vi "正面计算.vi"(0 "Image In":T1(plugin-control), 5 "图片处理效果参数":T13={"二值化参数"={"Lower value"=169.0, "Upper value"=255.0}, "形态学分析模式"=enum."Erode", "形态学 迭代次数"=3, "特殊分析-滤波"=[{"Measurement Parameter"=19, "Range Lower Value"=0.0, "Range Upper Value"=1400.0, "Range"=FALSE, "Measurement Type"=FALSE}], "特殊分析-移除/保留"=TRUE} {"特殊分析-滤波"."Measurement Parameter" items=["Center of Mass X", "Center of Mass Y", "First Pixel X", "First Pixel Y", "Bounding Rect Left", "Bounding Rect Top", "Bounding Rect Right", "Bounding Rect Bottom", "Max Feret Diameter Start X", "Max Feret Diameter Start Y", "Max Feret Diameter End X", "Max Feret Diameter End Y", "Max Horiz. Segment Length Left", "Max Horiz. Segment Length Right", "Max Horiz. Segment Length Row", "-", "Bounding Rect Width", "Bounding Rect Height", "Bounding Rect Diagonal", "Perimeter", "Convex Hull Perimeter", "Holes' Perimeter", "Max Feret Diameter", "Equivalent Ellipse Major Axis", "Equivalent Ellipse Minor Axis", "Equivalent Ellipse Minor Axis (Feret)", "Equivalent Rect Long Side", "Equivalent Rect Short Side", "Equivalent Rect Diagonal", "Equivalent Rect Short Side (Feret)", "Average Horiz. Segment Length", "Average Vert. Segment Length", "Hydraulic Radius", "Waddel Disk Diameter", "-", "Area", "Holes' Area", "Particle & Holes' Area", "Convex Hull Area", "Image Area", "-", "Number of Holes", "Number of Horiz. Segments", "Number of Vert. Segments", "-", "Orientation", "Max Feret Diameter Orientation", "-", "% Area/Image Area", "% Area/(Particle & Holes' Area)", "Ratio of Equivalent Ellipse Axes", "Ratio of Equivalent Rect Sides", "-", "Elongation Factor", "Compactness Factor", "Heywood Circularity Factor", "Type Factor", "-", "Sum X", "Sum Y", "Sum XX", "Sum XY", "Sum YY", "Sum XXX", "Sum XXY", "Sum XYY", "Sum YYY", "-", "Moment of Inertia XX", "Moment of Inertia XY", "Moment of Inertia YY", "Moment of Inertia XXX", "Moment of Inertia XXY", "Moment of Inertia XYY", "Moment of Inertia YYY", "Norm. Moment of Inertia XX", "Norm. Moment of Inertia XY", "Norm. Moment of Inertia YY", "Norm. Moment of Inertia XXX", "Norm. Moment of Inertia XXY", "Norm. Moment of Inertia XYY", "Norm. Moment of Inertia YYY", "Hu Moment 1", "Hu Moment 2", "Hu Moment 3", "Hu Moment 4", "Hu Moment 5", "Hu Moment 6", "Hu Moment 7"]}, 7 "定位分析参数设定":T12={"是否启动图片分析"=FALSE, "定位圆环ROI"={"Center X"=1247, "Center Y"=1475, "Inner Radius"=0, "Outer Radius"=400, "Start Angle"=0.0, "End Angle"=0.0}, "圆环Options "={"Process"=enum."Get First Edge", "Step Size"=10, "Max Pixel Radius"=3}, "Options (Find Circular)"={"Search  Direction"=1, "Edge Options"={"Edge Polarity"=0, "Kernel Size"=3, "Width"=3, "Minimum Edge Strength"=178.0, "Interpolation Type"=enum."Bilinear Fixed", "Data Processing Method"=enum."Average"}, "Show Search Area"=FALSE, "Show Search Lines"=FALSE, "Show Edges Found"=FALSE, "Show Result"=FALSE, "Search Area Color"=65280, "Search Lines Color"=255, "Edge Locations Color"=16776960, "Result Color"=16711680, "Overlay Group Name"=""}} {"Options (Find Circular)"."Search  Direction" items=["Outside to Inside", "Inside to Outside"]; "Options (Find Circular)"."Edge Options"."Edge Polarity" items=["All Edges", "Rising Edges", "Falling Edges"]; "Options (Find Circular)"."Edge Options"."Minimum Edge Strength" format="%.2f"; "Options (Find Circular)"."Edge Options"."Width" step=2; "Options (Find Circular)"."Edge Options"."Kernel Size" step=2; "定位圆环ROI"."End Angle" min=-90.0 max=90.0 step=1.0 format="%.2f"; "定位圆环ROI"."Start Angle" min=-90.0 max=90.0 step=1.0 format="%.2f"; "定位圆环ROI"."Center X" scale=0.0..1024.0}, 9 "分析参数设定":T9={"溢出距离下限"="", "溢出距离上限"="", "像素分辨率"="", "Search Direction "=enum."Annulus Outer To Inner", "Curve Extraction "={"Extraction Mode"=0, "Edge Threshold"=75, "Edge Filter Size"=0, "Min Length"=25, "Search Step Size"=15, "Max Endpoint Gap"=10, "Subpixel"=TRUE}, "Contour Selection "=enum."Closest To Search Start", "Curve Connection "=[{"Match Constraints"=0, "Min"=1.0, "Max"=12.0}], "Kernel Width "=5, "Curve Extraction 2 "={"Extraction Mode"=0, "Edge Threshold"=75, "Edge Filter Size"=0, "Min Length"=25, "Search Step Size"=15, "Max Endpoint Gap"=10, "Subpixel"=TRUE}, "Match Mode "={"Rotation"=FALSE, "Scale"=FALSE, "Occlusion"=FALSE}, "Smoothing Kernel "=0, "Template File Path "=path "C:/Users/hedongpo/Desktop/吕亚/Temp3.png", "Circle or Annulus"={"Center X"=1245, "Center Y"=1480, "Inner Radius"=238, "Outer Radius"=308, "Start Angle"=0.0, "End Angle"=0.0}} {"Circle or Annulus"."End Angle" min=-90.0 max=90.0 step=1.0 format="%.2f"; "Circle or Annulus"."Start Angle" min=-90.0 max=90.0 step=1.0 format="%.2f"; "Circle or Annulus"."Center X" scale=0.0..1024.0; "Curve Extraction"."Extraction Mode" items=["Normal", "Uniform Regions"]; "Curve Extraction"."Edge Filter Size" items=["Fine", "Normal", "Contour Tracing"]; "Curve Extraction"."Max Endpoint Gap" min=0; "Curve Extraction"."Search Step Size" min=1 max=255 step=1; "Curve Extraction"."Min Length" min=0; "Curve Extraction"."Edge Threshold" min=1 max=350 step=1; "Curve Connection"."Max" format="%.2f"; "Curve Connection"."Min" format="%.2f"; "Curve Connection"."Match Constraints" items=["Distance (pixel)", "Angle Difference (degrees)", "Connectivity Distance (pixel)", "Gradient Difference (degrees)"]; "Curve Extraction 2"."Extraction Mode" items=["Normal", "Uniform Regions"]; "Curve Extraction 2"."Edge Filter Size" items=["Fine", "Normal", "Contour Tracing"]; "Curve Extraction 2"."Max Endpoint Gap" min=0; "Curve Extraction 2"."Search Step Size" min=1 max=255 step=1; "Curve Extraction 2"."Min Length" min=0; "Curve Extraction 2"."Edge Threshold" min=1 max=350 step=1}, 11 "error in":errorcluster) -> (4 "Image Out":T1(plugin-control), 6 "Distances":T5(array[cluster]) {"Template Point"."Y" format="%.2f"; "Template Point"."X" format="%.2f"; "Target Point"."Y" format="%.2f"; "Target Point"."X" format="%.2f"}, 10 "Image Temple":T1, 15 "error out":errorcluster)   [LabVIEW 2017]
uses:
  <vilib>/vision/Measure.llb/Edge Options.ctl
  <vilib>/vision/Measure.llb/Edge Polarity.ctl
  <vilib>/vision/Contour.llb/IMAQ Contour Curve Extraction.ctl
  <vilib>/vision/Contour.llb/IMAQ Connect Range Setting.ctl
  <vilib>/vision/Image Controls.llb/IMAQ Image.ctl
  <vilib>/vision/Pattern Matching.llb/IMAQ Match Range Setting.ctl
  <vilib>/vision/NI_Vision_Development_Module.lvlib
panel:
  out "ROI Descriptor":T2 {"Contours"."Type" items=["No Selection", "Point", "Line", "Rectangle", "Oval", "Polygon", "Freehand Region", "Annulus", "Unused2", "Unused3", "Broken Line", "Freehand Line", "Rotated Rectangle"]}
  out "Coordinate System Out 2":T3 {"Measurement System"."Axis Reference" items=["Direct", "Indirect"]; "Measurement System"."Angle (deg)" format="%.2f"; "Measurement System"."Origin"."Y" format="%.2f"; "Measurement System"."Origin"."X" format="%.2f"; "Reference System"."Axis Reference" items=["Direct", "Indirect"]; "Reference System"."Angle (deg)" format="%.2f"; "Reference System"."Origin"."Y" format="%.2f"; "Reference System"."Origin"."X" format="%.2f"}
  out "Coordinate System Out":T3 {"Measurement System"."Axis Reference" items=["Direct", "Indirect"]; "Measurement System"."Angle (deg)" format="%.2f"; "Measurement System"."Origin"."Y" format="%.2f"; "Measurement System"."Origin"."X" format="%.2f"; "Reference System"."Axis Reference" items=["Direct", "Indirect"]; "Reference System"."Angle (deg)" format="%.2f"; "Reference System"."Origin"."Y" format="%.2f"; "Reference System"."Origin"."X" format="%.2f"}
  out "ROI Descriptor out 2":T2 {"Contours"."Type" items=["No Selection", "Point", "Line", "Rectangle", "Oval", "Polygon", "Freehand Region", "Annulus", "Unused2", "Unused3", "Broken Line", "Freehand Line", "Rotated Rectangle"]}
  out "输出簇":T4
  out "Center (Pixels) 2":cluster{"X":sgl, "Y":sgl}
  out "Valid?":bool
  out "Center (Pixels)":cluster{"X":sgl, "Y":sgl}
  out "ROI Descriptor out":T2 {"Contours"."Type" items=["No Selection", "Point", "Line", "Rectangle", "Oval", "Polygon", "Freehand Region", "Annulus", "Unused2", "Unused3", "Broken Line", "Freehand Line", "Rotated Rectangle"]}
  in  "File Path":path
  # "Range"
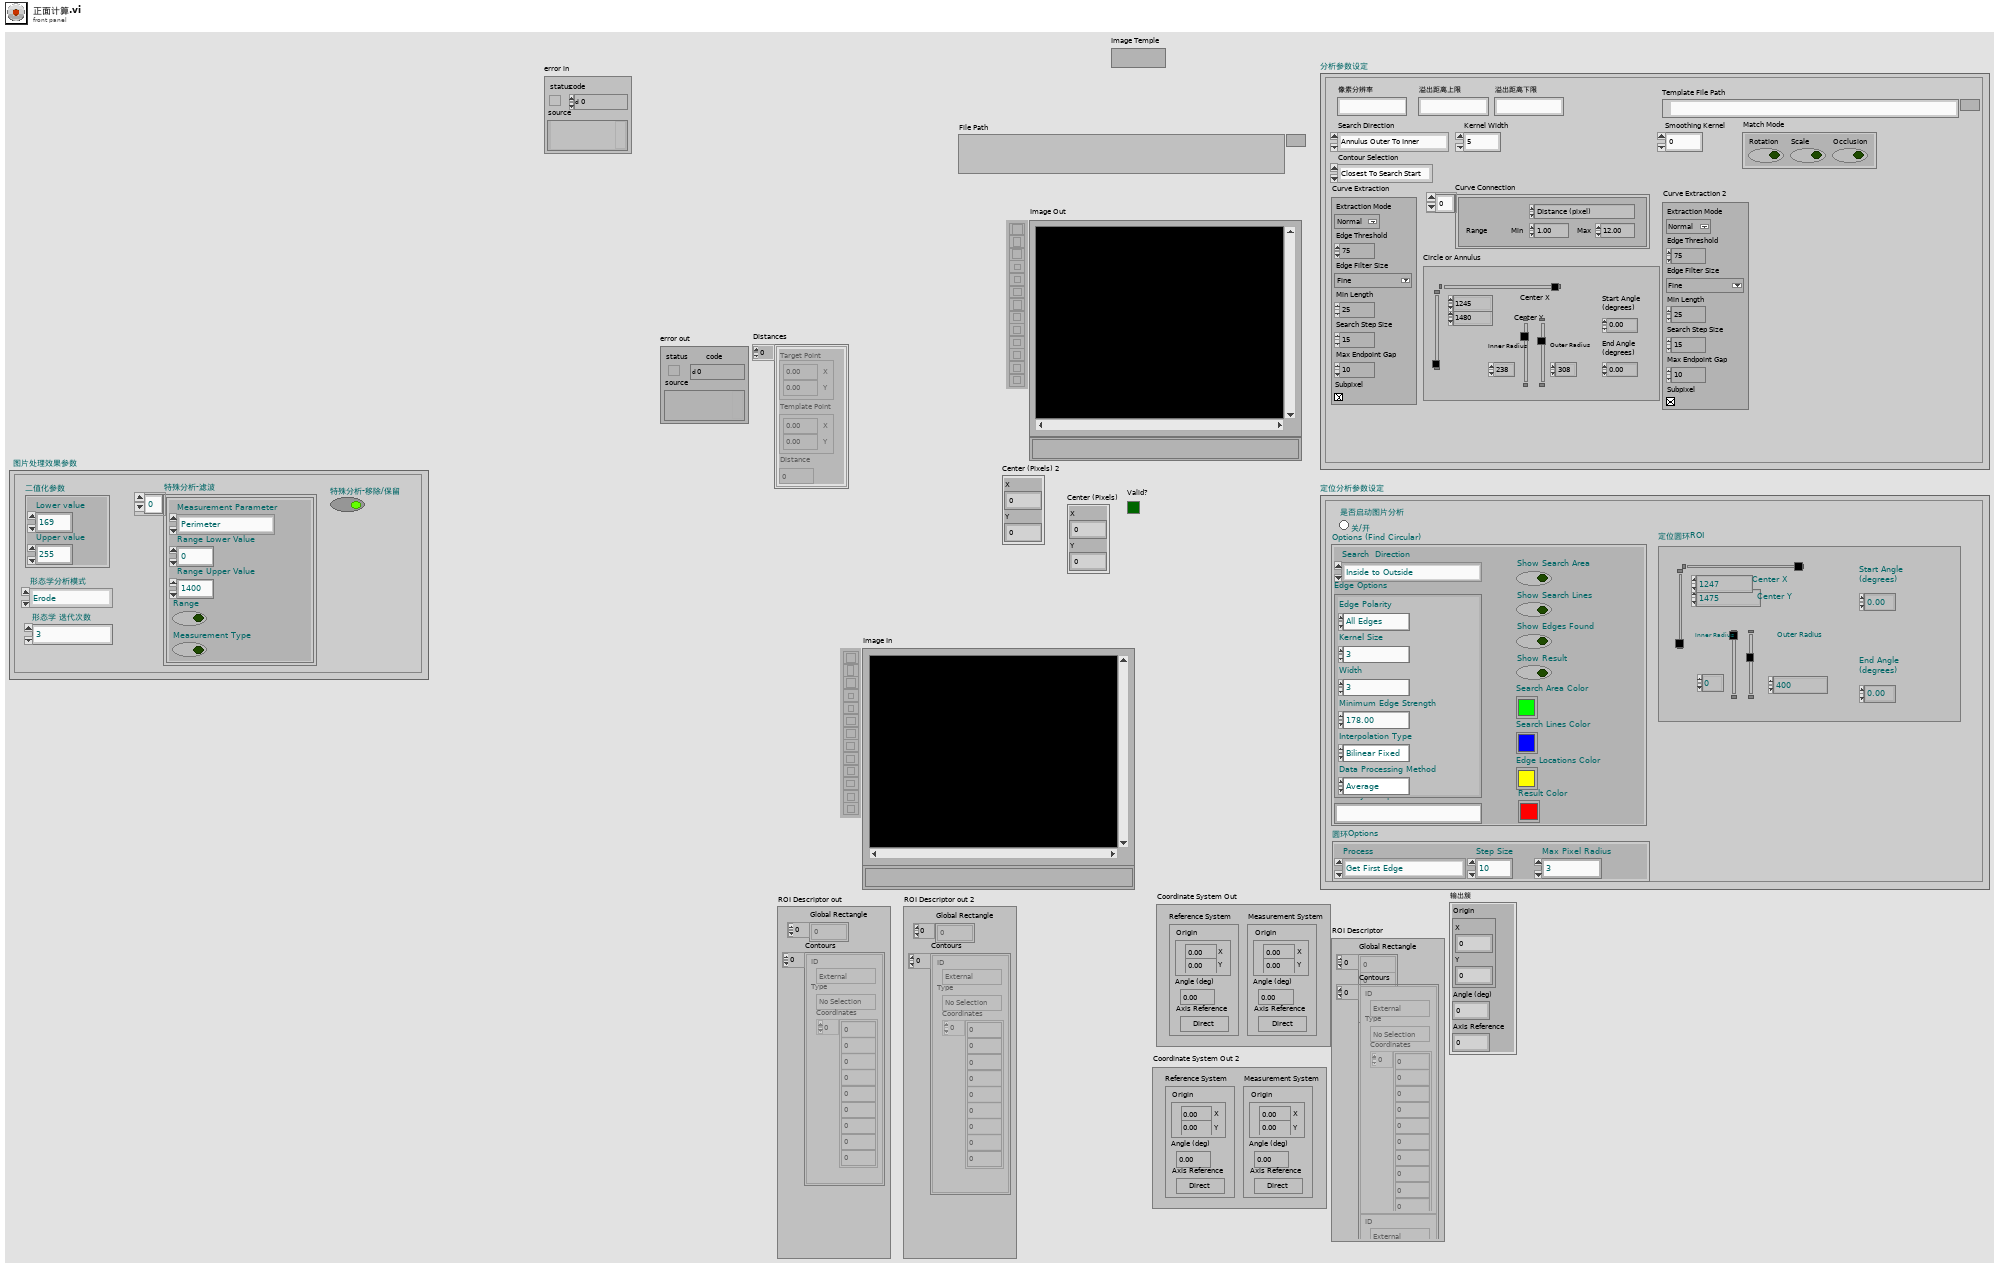
[diagram p1: front panel]
types:
  T1 = typedef "IMAQ Image.ctl" = refnum<image>
  T2 = typedef "ROI Descriptor" = cluster{"Global Rectangle":i32[], "Contours":cluster{"ID":enum32{"External", "Internal"}, "Type":u32, "Coordinates":i32[]}[]}
  T3 = typedef "IMAQ Coordinate System" = cluster{"Reference System":cluster{"Origin":cluster{"X":sgl, "Y":sgl}, "Angle (deg)":sgl, "Axis Reference":u32}, "Measurement System":cluster{"Origin":cluster{"X":sgl, "Y":sgl}, "Angle (deg)":sgl, "Axis Reference":u32}}
  T4 = cluster{"Origin":cluster{"X":sgl, "Y":sgl}, "Angle (deg)":sgl, "Axis Reference":u32}
  T5 = cluster{"Target Point":cluster{"X":dbl, "Y":dbl}, "Template Point":cluster{"X":dbl, "Y":dbl}, "Distance":dbl}[]
  T6 = typedef "IMAQ Contour Curve Extraction.ctl" = cluster{"Extraction Mode":u32, "Edge Threshold":i32, "Edge Filter Size":u32, "Min Length":i32, "Search Step Size":i32, "Max Endpoint Gap":i32, "Subpixel":bool}
  T7 = typedef "IMAQ Connect Range Setting.ctl" = cluster{"Match Constraints":u32, "Min":dbl, "Max":dbl}
  T8 = typedef "IMAQ Circle" = cluster{"Center X":i32, "Center Y":i32, "Inner Radius":i32, "Outer Radius":i32, "Start Angle":dbl, "End Angle":dbl}
  T9 = cluster{"溢出距离下限":string, "溢出距离上限":string, "像素分辨率":string, "Search Direction ":enum16{"Rect Left To Right", "Rect Right To Left", "Rect Top To Bottom", "Rect Bottom To Top", "Annulus Inner To Outer", "Annulus Outer To Inner", "Annulus Start Angle To End Angle", "Annulus End Angle To Start Angle"}, "Curve Extraction ":T6, "Contour Selection ":enum16{"Closest To Search Start", "Maximum Length", "Strongest Mean Gradient Change"}, "Curve Connection ":T7[], "Kernel Width ":u32, "Curve Extraction 2 ":T6, "Match Mode ":cluster{"Rotation":bool, "Scale":bool, "Occlusion":bool}, "Smoothing Kernel ":u32, "Template File Path ":path, "Circle or Annulus":T8}
  T10 = typedef "Edge Options.ctl" = cluster{"Edge Polarity":T11, "Kernel Size":u32, "Width":u32, "Minimum Edge Strength":sgl, "Interpolation Type":enum32{"Zero Order", "Bilinear", "Quadratic", "Cubic", "Bilinear Fixed"}, "Data Processing Method":enum32{"Average", "Median"}}
  T11 = typedef "Edge Polarity.ctl" = u32
  T12 = cluster{"是否启动图片分析":bool, "定位圆环ROI":T8, "圆环Options ":cluster{"Process":enum16{"Get First Edge", "Get First + Last Edge", "Get All Edges", "Get Best Edge"}, "Step Size":i32, "Max Pixel Radius":i32}, "Options (Find Circular)":cluster{"Search  Direction":u32, "Edge Options":T10, "Show Search Area":bool, "Show Search Lines":bool, "Show Edges Found":bool, "Show Result":bool, "Search Area Color":u32, "Search Lines Color":u32, "Edge Locations Color":u32, "Result Color":u32, "Overlay Group Name":string}}
  T13 = cluster{"二值化参数":cluster{"Lower value":sgl, "Upper value":sgl}, "形态学分析模式":enum32{"AutoM", "Close", "Dilate", "Erode", "Gradient", "Gradient out", "Gradient in", "Hit miss", "Open", "PClose", "POpen", "Thick", "Thin"}, "形态学 迭代次数":i32, "特殊分析-滤波":cluster{"Measurement Parameter":i32, "Range Lower Value":dbl, "Range Upper Value":dbl, "Range":bool, "Measurement Type":bool}[], "特殊分析-移除/保留":bool}
  T14 = cluster{"Overlay?":bool, "Color":u32, "Width":u32, "Maintain Width?":bool}
  T15 = cluster{"Search  Direction":u32, "Edge Options":T10, "Show Search Area":bool, "Show Search Lines":bool, "Show Edges Found":bool, "Show Result":bool, "Search Area Color":u32, "Search Lines Color":u32, "Edge Locations Color":u32, "Result Color":u32, "Overlay Group Name":string}
  T16 = typedef "IMAQ Match Range Setting.ctl" = cluster{"Match Constraints":u32, "Min":dbl, "Max":dbl}
  T17 = cluster{"Setup Data Item":u16, "Item Value":dbl}[]
  T18 = cluster{"Rotation":bool, "Scale":bool, "Occlusion":bool}
  T19 = enum16{"Closest To Search Start", "Maximum Length", "Strongest Mean Gradient Change"}
  T20 = enum16{"Rect Left To Right", "Rect Right To Left", "Rect Top To Bottom", "Rect Bottom To Top", "Annulus Inner To Outer", "Annulus Outer To Inner", "Annulus Start Angle To End Angle", "Annulus End Angle To Start Angle"}
  T21 = enum16{"Reset", "Update Coordinate System", "Get Coordinate System"}
  T22 = enum16{"Horizontal Motion", "Vertical Motion", "Horizontal and Vertical Motion", "Horizontal, Vertical and Angular Motion"}
  T23 = cluster{"Process":enum16{"Get First Edge", "Get First + Last Edge", "Get All Edges", "Get Best Edge"}, "Step Size":i32, "Max Pixel Radius":i32}
  T24 = cluster{"Global Rectangle":i32[], "Contours":cluster{"ID":enum32{"External", "Internal"}, "Type":u32, "Coordinates":i32[]}[]}
  T25 = cluster{"Measurement Parameter":i32, "Range Lower Value":dbl, "Range Upper Value":dbl, "Range":bool, "Measurement Type":bool}[]
  T26 = enum32{"AutoM", "Close", "Dilate", "Erode", "Gradient", "Gradient out", "Gradient in", "Hit miss", "Open", "PClose", "POpen", "Thick", "Thin"}
  T27 = typedef "Image Type" = u32
  T28 = cluster{"histogram":u32[], "Minimal Value":sgl, "Maximal Value":sgl, "Starting Value":sgl, "Interval Width":sgl, "Mean Value":sgl, "Standard  Variation":sgl, "Area (pixels)":i32}
  T29 = cluster{"Center (Pixels)":cluster{"X":sgl, "Y":sgl}, "Radius (Pixels)":dbl, "Center (Real-World)":cluster{"X":sgl, "Y":sgl}, "Radius (Real-World)":dbl, "Roundness (Real-World)":dbl, "Average Strength":dbl, "Average SNR (dB)":dbl}
  T30 = cluster{"Left":i32, "Top":i32, "Right":i32, "Bottom":i32}
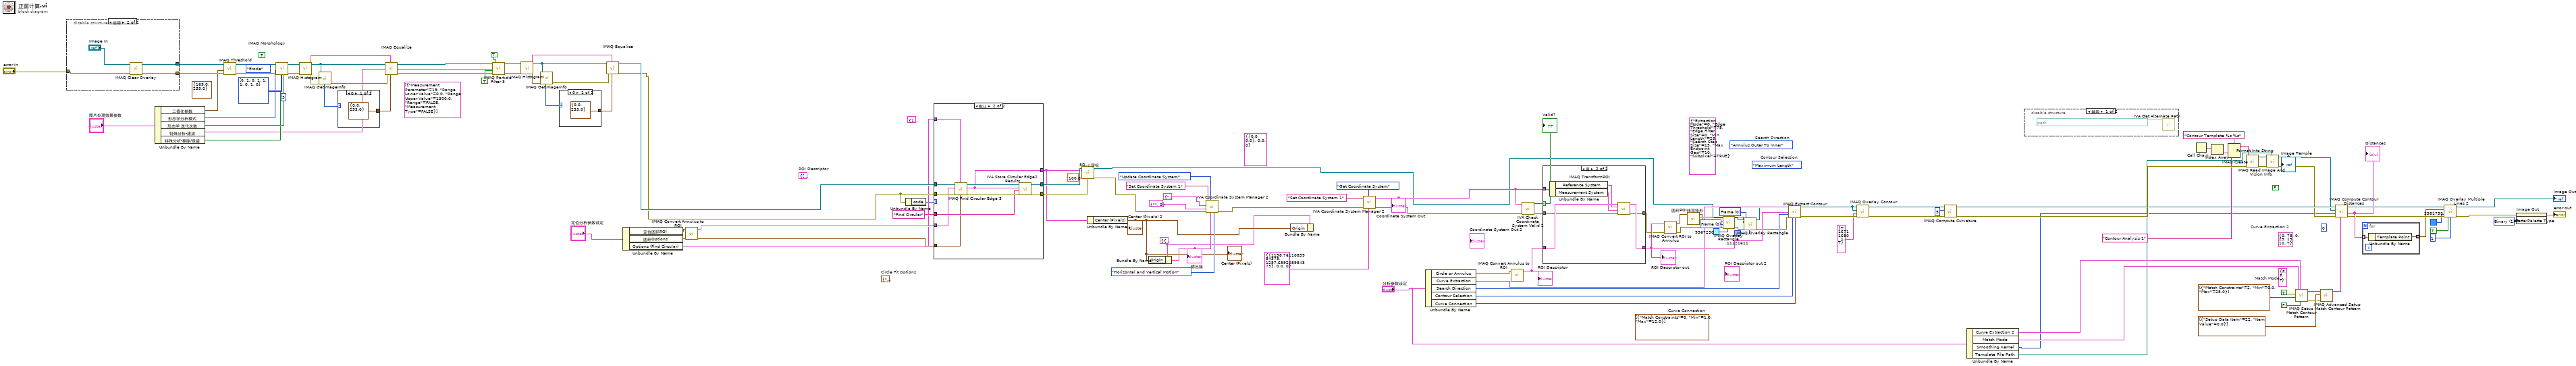
[diagram p0: block diagram]
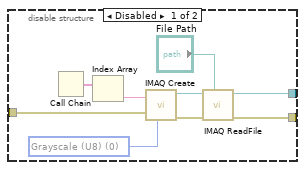
[diagram p2: hidden frame]
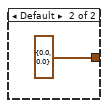
[diagram p6: hidden frame]
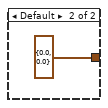
[diagram p7: hidden frame]
diagram:
  (unwired) FALSE
  w16 = u32 0 items=["Frame", "Fill", "Highlight"] ("Drawing Mode (Frame)")
  w19 = u32 0 items=["Frame", "Fill", "Highlight"] ("Drawing Mode (Frame)")
  (unwired) T6 {"Extraction Mode"=0, "Edge Threshold"=75, "Edge Filter Size"=0, "Min Length"=25, "Search Step Size"=15, "Max Endpoint Gap"=10, "Subpixel"=TRUE} ("Curve Extraction")
  (unwired) T15 {"Search  Direction"=1, "Edge Options"={"Edge Polarity"=0, "Kernel Size"=3, "Width"=3, "Minimum Edge Strength"=178.0, "Interpolation Type"=enum."Bilinear Fixed", "Data Processing Method"=enum."Average"}, "Show Search Area"=TRUE, "Show Search Lines"=TRUE, "Show Edges Found"=TRUE, "Show Result"=TRUE, "Search Area Color"=65280, "Search Lines Color"=255, "Edge Locations Color"=16776960, "Result Color"=16711680, "Overlay Group Name"=""} ("Options")
  (unwired) T6 {"Extraction Mode"=0, "Edge Threshold"=75, "Edge Filter Size"=0, "Min Length"=25, "Search Step Size"=15, "Max Endpoint Gap"=10, "Subpixel"=TRUE}  # Curve Extraction 2
  (unwired) T18 {"Rotation"=FALSE, "Scale"=FALSE, "Occlusion"=FALSE}  # Match Mode
  (unwired) u32 0 ("Smoothing Kernel")
  (unwired) T7[] [{"Match Constraints"=0, "Min"=1.0, "Max"=12.0}]  # Curve Connection
  (unwired) T19."Maximum Length"  # Contour Selection
  (unwired) T20."Annulus Outer To Inner"  # Search Direction
  (unwired) T4 {"Origin"={"X"=0.0, "Y"=0.0}, "Angle (deg)"=0.0, "Axis Reference"=0} ("Reference System")
  w2 = T4 {"Origin"={"X"=0.0, "Y"=0.0}, "Angle (deg)"=0.0, "Axis Reference"=0} ("Reference System")
  (unwired) T23 {"Process"=enum."Get First Edge", "Step Size"=20, "Max Pixel Radius"=3}  # Circle Fit Options
  (unwired) T24 {"Global Rectangle"=[683, 713, 1453, 1482], "Contours"=[{"ID"=enum."External", "Type"=7, "Coordinates"=[1067, 1097, 71, 384, 0, 0]}]}  # ROI Descriptor
  w96 = u32 1 items=["Grayscale", "Binary", "Gradient", "Rainbow", "Temperature", "User Defined", "Binary 16 Bit", "Gradient 16 Bit", "Rainbow 16 Bit", "Temperature 16 Bit", "User Defined 16 Bit"] ("Palette Type")
  (unwired) T25 [{"Measurement Parameter"=19, "Range Lower Value"=0.0, "Range Upper Value"=1300.0, "Range"=FALSE, "Measurement Type"=FALSE}] ("Selection Values")
  (unwired) 3 ("Number of iterations (1)")
  (unwired) T26."Erode" ("Operation")
  (unwired) FALSE ("Square/Hexa (Square)")
  (unwired) cluster{"Lower value":sgl, "Upper value":sgl} {"Lower value"=169.0, "Upper value"=255.0} ("Range")
  n1 = disable-structure shown="启用" {
    disable-tunnel: [w130 w131] -> w121
    disable-tunnel: "error in" -> [w127 w132]
    disable-tunnel: [w123 w133] -> w119
    frame Disabled {
      w124 = T27 0 items=["Grayscale (U8)", "Grayscale (I16)", "Grayscale (SGL)", "Complex (CSG)", "RGB (U32)", "HSL (U32)", "RGB (U64)", "Grayscale (U16)"] ("Image Type")
      n2 = Call Chain() -> (call chain=w126:string[])
      n3 = Index Array(array=w126) -> (element=w125:string)  [unwired: 1 in]
      n4 = call "IMAQ Create"("Image Name"=w125, "Image Type"=w124, "error in (no error)"=w127) -> ("New Image"=w129:T1, "error out"=w128:errorcluster)  [unwired: 1 in, 1 out]
      n5 = call "IMAQ ReadFile"("File Path"="File Path", "error in (no error)"=w128, "Image"=w129) -> ("error out"=w130:errorcluster, "Image Out"=w123:T1)  [unwired: 2 in, 5 out]
    }
    frame Enabled {
      n6 = call "IMAQ Clear Overlay"("error in (no error)"=w132, "Image"="Image In") -> ("error out"=w131:errorcluster, "Image Out"=w133:T1)  [unwired: 8 in]
    }
  }
  n7 = Unbundle By Name("图片处理效果参数") -> ("二值化参数"=w94:cluster{"Lower value":sgl, "Upper value":sgl}, "形态学分析模式"=w93:T26, "形态学 迭代次数"=w92:i32, "特殊分析-滤波"=w90:T25, "特殊分析-移除/保留"=w91:bool)
  n8 = call "IMAQ Threshold"("error in (no error)"=w121, "Range"=w94, "Image Src"=w119) -> ("error out"=w118:errorcluster, "Image Dst Out"=w116:T1)  [unwired: 3 in, 4 out]
  n9 = call "IMAQ Morphology"("Number of iterations (1)"=w92, "Structuring Element"=i32[][] [[0, 1, 0], [1, 1, 1], [0, 1, 0]], "Square/Hexa (Square)"=w91, "error in (no error)"=w118, "Operation"=w93, "Image Src"=w116) -> ("error out"=w115:errorcluster, "Image Dst Out"=w111:T1)  [unwired: 1 in, 3 out]
  n10 = call "IMAQ Histogram"("error in (no error)"=w115, "Image"=w111) -> ("error out"=w110:errorcluster, "Histogram Report"=w113:T28)  [unwired: 3 in, 5 out]
  n11 = call "IMAQ GetImageInfo"("error in (no error)"=w110, "Image"=w111) -> ("error out"=w109:errorcluster, "Image Type"=w112:T27)  [unwired: 8 out]
  n12 = case "条件结构" shown="0" w112 {
    tunnel: [cluster{"Minimum":sgl, "Maximum":sgl} {"Minimum"=0.0, "Maximum"=255.0} ("Range") cluster{"Minimum":sgl, "Maximum":sgl} {"Minimum"=0.0, "Maximum"=0.0} ("Range")] -> w108
    frame 0 {
    }
    frame Default {
    }
  }
  n13 = call "IMAQ Equalize"("Range"=w108, "Histogram Report"=w113, "error in (no error)"=w109, "Image Src"=w111) -> ("error out"=w114:errorcluster, "Image Dst Out"=w104:T1)  [unwired: 2 in, 4 out]
  n14 = call "IMAQ Particle Filter 3"("Image Src"=w104, "Connectivity 4/8 (8)"=TRUE, "Selection Values"=w90, "Keep/Remove Particles (F)"=TRUE ("Keep/Remove Particles"), "error in (no error)"=w114) -> ("Image Dst Out"=w101:T1, "error out"=w105:errorcluster)  [unwired: 4 in, 5 out]
  n15 = call "IMAQ Histogram"("error in (no error)"=w105, "Image"=w101) -> ("error out"=w100:errorcluster, "Histogram Report"=w103:T28)  [unwired: 3 in, 5 out]
  n16 = call "IMAQ GetImageInfo"("error in (no error)"=w100, "Image"=w101) -> ("error out"=w99:errorcluster, "Image Type"=w102:T27)  [unwired: 8 out]
  n17 = case "条件结构" shown="0" w102 {
    tunnel: [cluster{"Minimum":sgl, "Maximum":sgl} {"Minimum"=0.0, "Maximum"=255.0} ("Range") cluster{"Minimum":sgl, "Maximum":sgl} {"Minimum"=0.0, "Maximum"=0.0} ("Range")] -> w98
    frame 0 {
    }
    frame Default {
    }
  }
  n18 = call "IMAQ Equalize"("Range"=w98, "Histogram Report"=w103, "error in (no error)"=w99, "Image Src"=w101) -> ("error out"=w51:errorcluster, "Image Dst Out"=w52:T1)  [unwired: 2 in, 4 out]
  n19 = Unbundle By Name("定位分析参数设定") -> ("定位圆环ROI"=w47:T8, "圆环Options"=w45:T23, "Options (Find Circular)"=w44:T15)
  n20 = call "IMAQ Convert Annulus to ROI"("Annulus"=w47) -> ("ROI Descriptor"=w46:T2)  [unwired: 8 in, 1 out]
  n21 = Unbundle By Name(w51) -> ("code"=w88:i32)
  n22 = case "条件结构" shown="默认" w88 {
    tunnel: w44 -> [_ w140]
    tunnel: w52 -> [w139 w150]
    tunnel: w51 -> [_ w149]
    tunnel: [_ w147] -> w42
    tunnel: [w139 w145] -> w43
    tunnel: "Find Circular" ("Step Name") -> [_ w144]
    tunnel: w46 -> [_ w143]
    tunnel: w45 -> [_ w142]
    tunnel: [_ w141] -> w39
    frame -1074396199, -1074396198 {
      # "Discard Coordinate System Error"
    }
    frame Default {
      n23 = call "IMAQ Find Circular Edge 3"("Circle Fit Options"=w142, "Options"=w140, "error in (no error)"=w149, "ROI Descriptor"=w143, "Image"=w150) -> ("error out"=w148:errorcluster, "Fitted Circle"=w141:T29, "Image Out"=w146:T1)  [unwired: 2 in, 2 out]
      n24 = call <vilib>:"IVA Store Circular Edge2 Results.vi"("error in (no error)"=w148, "Step Name"=w144, "Fitted Circle"=w141, "Image in"=w146) -> ("error out"=w147:errorcluster, "Image dup"=w145:T1)  [unwired: 2 in, 4 out]
    }
  }
  n25 = call "3D-十字标.vi"("error in (no error)"=w42, "radius"=100.0, "Fitted Circle (Find Circular)"=w39, "输入图片"=w43) -> ("error out"=w41:errorcluster, "输出图片"=w27:T1)  [unwired: 6 in]
  n26 = Unbundle By Name(w39) -> ("Center (Pixels)"=w32:cluster{"X":sgl, "Y":sgl})
  "Center (Pixels)" <- w32
  "Center (Pixels) 2" <- w32
  n27 = Bundle By Name(cluster=w2, "Origin"=w32) -> (w31:T4)
  "输出簇" <- w31
  n28 = call <vilib>:"IVA Coordinate System Manager 2.vi"("Mode"=T22."Horizontal and Vertical Motion", "Reference System"=w31, "Function"=T21."Update Coordinate System", "error in (no error)"=w41, "Angle ID"=cluster{"GUID":string, "Index":i32} {"GUID"="", "Index"=0}, "Origin ID"=cluster{"GUID":string, "Index":i32} {"GUID"="Find Circular", "Index"=0}, "Coordinate System Name"="Set Coordinate System 1") -> ("error out"=w84:errorcluster)  [unwired: 4 out]
  n29 = Bundle By Name(cluster=w2, "Origin"=w32) -> ()  [unwired: 1 out]
  n30 = call <vilib>:"IVA Coordinate System Manager 2.vi"("Reference System"=T4 {"Origin"={"X"=1198.7611, "Y"=1257.6892}, "Angle (deg)"=0.0, "Axis Reference"=0}, "Function"=T21."Get Coordinate System", "error in (no error)"=w84, "Coordinate System Name"="Set Coordinate System 1") -> ("error out"=w81:errorcluster, "Coordinate System Out"=w80:T3)  [unwired: 3 in, 3 out]
  "Coordinate System Out" <- w80
  n31 = Unbundle By Name("分析参数设定") -> ("Circle or Annulus"=w38:T8, "Curve Extraction"=w37:T6, "Search Direction"=w36:T20, "Contour Selection"=w35:T19, "Curve Connection"=w34:T7[])
  n32 = call "IMAQ Convert Annulus to ROI"("Annulus"=w38) -> ("ROI Descriptor"=w33:T2)  [unwired: 8 in, 1 out]
  "ROI Descriptor" <- w33
  n33 = call <vilib>:"IVA Check Coordinate System Valid 2.vi"("error in (no error)"=w81, "Coordinate System"=w80) -> ("error out"=w78:errorcluster, "Valid?"=w79:bool)  [unwired: 8 out]
  "Valid?" <- w79
  n34 = case "条件结构" shown="真" w79 {
    tunnel: w33 -> [w152 w159]
    tunnel: [w152 w156] -> w30
    tunnel: [w151 w155] -> w29
    tunnel: w80 -> [_ w154]
    tunnel: w78 -> [w151 w153]
    frame False {
    }
    frame True {
      n35 = Unbundle By Name(w154) -> ("Reference System"=w158:T4, "Measurement System"=w157:T4)
      n36 = call "IMAQ TransformROI"("error in (no error)"=w153, "New Reference"=w157, "Base Reference"=w158, "ROI Descriptor"=w159) -> ("error out"=w155:errorcluster, "ROI Descriptor out"=w156:T2)  [unwired: 6 out]
    }
  }
  "ROI Descriptor out" <- w30
  n37 = call "IMAQ Convert ROI to Annulus"("error in (no error)"=w29, "ROI Descriptor"=w30) -> ("error out"=w25:errorcluster, "Annulus"=w22:T8)  [unwired: 7 in]
  n38 = call "圆环ROI转双矩形.vi"("Annulus 2"=w22) -> ("内环"=w20:T30, "外环"=w21:T30)  [unwired: 9 in]
  n39 = call "IMAQ Overlay Rectangle"("Color"=u32 9567230, "error in (no error)"=w25, "Drawing Mode (Frame)"=w19, "Rectangle"=w21, "Image"=w27) -> ("error out"=w24:errorcluster, "Image Out"=w28:T1)  [unwired: 5 in]
  n40 = call "IMAQ Overlay Rectangle"("Color"=u32 11121611, "error in (no error)"=w24, "Drawing Mode (Frame)"=w16, "Rectangle"=w20, "Image"=w28) -> ("error out"=w23:errorcluster, "Image Out"=w26:T1)  [unwired: 5 in]
  n41 = call "IMAQ Extract Contour"("Source Image"=w26, "Curve Extraction"=w37, "ROI Descriptor"=w30, "Search Direction"=w36, "error in (no error)"=w23, "Contour Selection"=w35, "Curve Connection"=w34) -> ("Source Image Out"=w74:T1, "error out"=w77:errorcluster)  [unwired: 1 in, 6 out]
  n42 = call "IMAQ Overlay Contour"("error in (no error)"=w77, "Contour Points Settings"=T14 {"Overlay?"=TRUE, "Color"=16711680, "Width"=1, "Maintain Width?"=TRUE}, "Contour Image"=w74, "Image"=w74) -> ("error out"=w75:errorcluster, "Image Out"=w73:T1)  [unwired: 2 in, 4 out]
  n43 = call "IMAQ Compute Curvature"("error in (no error)"=w75, "Kernel Width"=u32 5, "Contour Image"=w73) -> ("error out"=w72:errorcluster, "Contour Image Out (dup)"=w69:T1)  [unwired: 1 in, 6 out]
  n44 = Unbundle By Name("分析参数设定") -> ("Curve Extraction 2"=w14:T6, "Match Mode"=w13:T18, "Smoothing Kernel"=w12:u32, "Template File Path"=w5:path)
  n45 = disable-structure shown="禁用" {
    frame Disabled {
      n46 = call <vilib>:"IVA Get Alternate Path.vi"("Path In"=path "C:/Users/hedongpo/Desktop/吕亚/Temp3.png" ("Template File Path")) -> ()  [unwired: 11 out]
    }
    frame Enabled {
    }
  }
  n47 = Call Chain() -> (call chain=w9:string[])
  n48 = Index Array(array=w9) -> (element=w8:string)  [unwired: 1 in]
  n49 = Format Into String(format string="Contour Template %s %s" ("Image Name"), w8, "Contour Analysis 1" ("Step Name")) -> (resulting string=w11:string)  [unwired: 2 in, 1 out]
  n50 = call "IMAQ Create"("Image Name"=w11, "error in (no error)"=w72) -> ("New Image"=w7:T1, "error out"=w6:errorcluster)  [unwired: 2 in, 1 out]
  n51 = call "IMAQ Read Image And Vision Info"("File Path"=w5, "error in (no error)"=w6, "Image"=w7) -> ("error out"=w67:errorcluster, "Image Out"=w68:T1)  [unwired: 1 in, 6 out]
  "Image Temple" <- w68
  n52 = call "IMAQ Setup Match Contour Pattern"("Use Learn Curve Extraction"=FALSE, "Curve Extraction"=w14, "Range Settings"=T16[] [{"Match Constraints"=2, "Min"=0.0, "Max"=25.0}], "Subpixel Accuracy"=TRUE, "Match Mode"=w13) -> ("error out"=w53:errorcluster, "Match Contour Pattern Setup Data"=w57:string)  [unwired: 1 in, 4 out]
  n53 = call "IMAQ Advanced Setup Match Contour Pattern"("Match Contour Pattern Setup Data In"=w57, "Advanced Contour Match Options"=T17 [{"Setup Data Item"=22, "Item Value"=0.0}], "error in (no error)"=w53) -> ("Match Contour Pattern Setup Data Out"=w56:string)  [unwired: 7 out]
  n54 = call "IMAQ Compute Contour Distances"("Match Contour Pattern Setup Data"=w56, "error in (no error)"=w67, "Smoothing Kernel"=w12, "Template Contour Image"=w68, "Target Contour Image"=w69) -> ("error out"=w62:errorcluster, "Distances"=w64:T5, "Target Contour Image Out (dup)"=w63:T1)  [unwired: 4 out]
  "Distances" <- w64
  n55 = for "For循环" {
    tunnel: w64 -> [w162] mode=indexing
    tunnel: [w161] -> w61 mode=indexing
    n56 = Unbundle By Name(w162) -> ("Template Point"=w161:cluster{"X":dbl, "Y":dbl})
  }
  n57 = call "IMAQ Overlay Multiple Lines 2"("Image"=w63, "Line End Points"=w61, "Color"=u32 3381759, "error in (no error)"=w62, "Maintain Width?"=TRUE, "Width"=u32 1) -> ("Image Out"=→"Image Out":T1, "error out"=w49:errorcluster)  [unwired: 2 in, 6 out]
  n58 = property on="Image Out" class="ImageControl"(error in=w49, "Palette:Palette Type"=w96) -> (error out=→"error out":errorcluster)  [unwired: 1 in, 1 out]
